vi "Check If Valid response.vi"(0 "string":string, 1 "error in (no error)":errorcluster) -> (18 "Valid":bool, 20 "string out":string, 21 "error out":errorcluster)   [LabVIEW 2020]
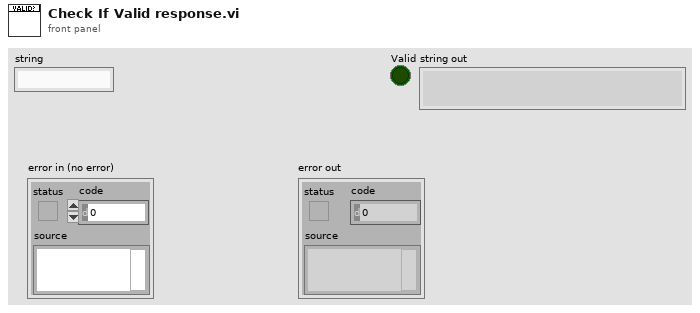
[diagram p1: front panel]
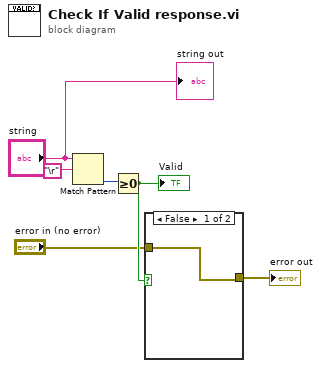
[diagram p0: block diagram]
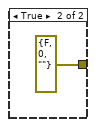
[diagram p2: hidden frame]
diagram:
  n1 = Match Pattern(string="string", regular expression="\r") -> (offset past match=w4:i32)  [unwired: 1 in, 3 out]
  n2 = Greater Or Equal To 0?(x=w4) -> (x >= 0?=w3:bool)
  "Valid" <- w3
  n3 = case shown="False" w3 {
    tunnel: [w7 errorcluster {"status"=FALSE, "code"=0, "source"=""} ("error out")] -> w2
    tunnel: "error in (no error)" -> [w7 _]
    frame False {
    }
    frame True {
    }
  }
  "error out" <- w2
  "string out" <- "string"
